vi "Main.vi"() -> ()   [LabVIEW 2019]
uses:
  <vilib>/addons/WireFlow/_WireQueue/MQTT API/MQTT_API.lvclass
panel:
  in  "stop":bool
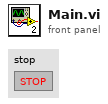
[diagram p1: front panel]
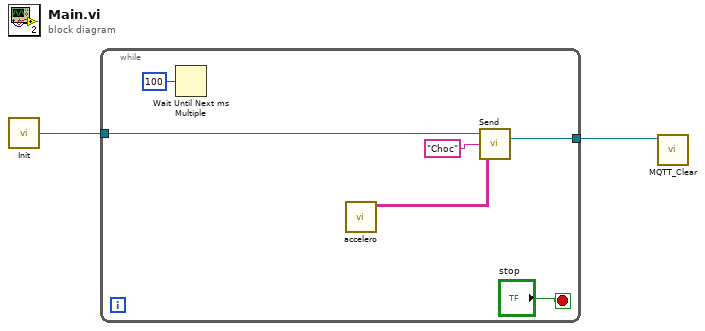
[diagram p0: block diagram]
diagram:
  n1 = call "Init.vi"() -> ("MQTT_API out"=w2:refnum<class "MQTT_API.lvclass">)
  n2 = while {
    tunnel: w2 -> [w7]
    tunnel: [w5] -> w1
    stop <- "stop" stop-if-true
    n3 = Wait Until Next ms Multiple(millisecond multiple=u32 100) -> ()  [unwired: 1 out]
    n4 = call "accelero.vi"() -> ("output array"=w3:string[][])  [unwired: 11 in]
    n5 = call "Send.vi"("Array"=w3, "Topic"="Choc", "MQTT_API in"=w7) -> ("MQTT_API out"=w5:refnum<class "MQTT_API.lvclass">)
  }
  n6 = call <vilib>:"MQTT_Clear.vi"("MQTT_API in"=w1) -> ()  [unwired: 9 in, 2 out]
